vi "Get Probe Control Params.vi"(11 "Probe Select":i32) -> (1 "Integ Count":u16, 2 "Laser Gain":u8, 3 "Laser Init Pwr":u16)   [LabVIEW 2015, in "Tool Cfg.lvlib"]
uses:
  Tool Cfg.lvlib
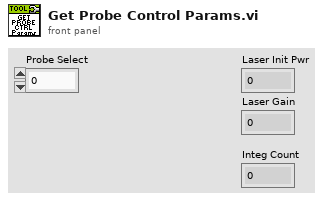
[diagram p1: front panel]
types:
  T1 = typedef "Tool Cfg.lvlib/_ProbeConfigParams Cluster--typedef.ctl" = cluster{"Name":string, "Laser Init Pwr":u16, "Laser Gain":u8, "Integ Count":u16, "Meas. Range":sgl, "Angle":sgl, "Probe Offset":sgl, "Sensor Block":T2}
  T2 = typedef "Tool Cfg.lvlib/_Sensor Block Cluster--typedef.ctl" = cluster{"nSensors":u16, "SensorCfgParams Array":T3[]}
  T3 = typedef "Tool Cfg.lvlib/_SensorConfigParams Cluster--typedef.ctl" = cluster{"Total Pixels":u16, "Positive  Peaks":bool, "CalibrCoefArray":dbl[], "Start Idx":u16, "End Idx":u16}
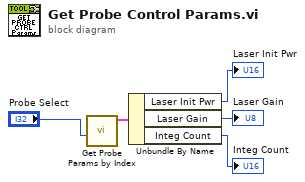
[diagram p0: block diagram]
diagram:
  n1 = call "Get Probe Params by Index.vi"("Probe Select"="Probe Select") -> ("Probe Cfg Params"=w5:T1)  [unwired: 10 in]
  n2 = Unbundle By Name(w5) -> ("Laser Init Pwr"=→"Laser Init Pwr":u16, "Laser Gain"=→"Laser Gain":u8, "Integ Count"=→"Integ Count":u16)
